vi "Draw Staff.vi"(4 "Line Spacing":i16=30, 6 "Line Length":i16=600, 9 "Start y":i16=200, 10 "Start x":i16=80, 11 "picture in":picture) -> (1 "End y":i16=230, 3 "picture out":picture)   [LabVIEW 2014]
panel:
  in  "y":i16=-120
  in  "x":i16
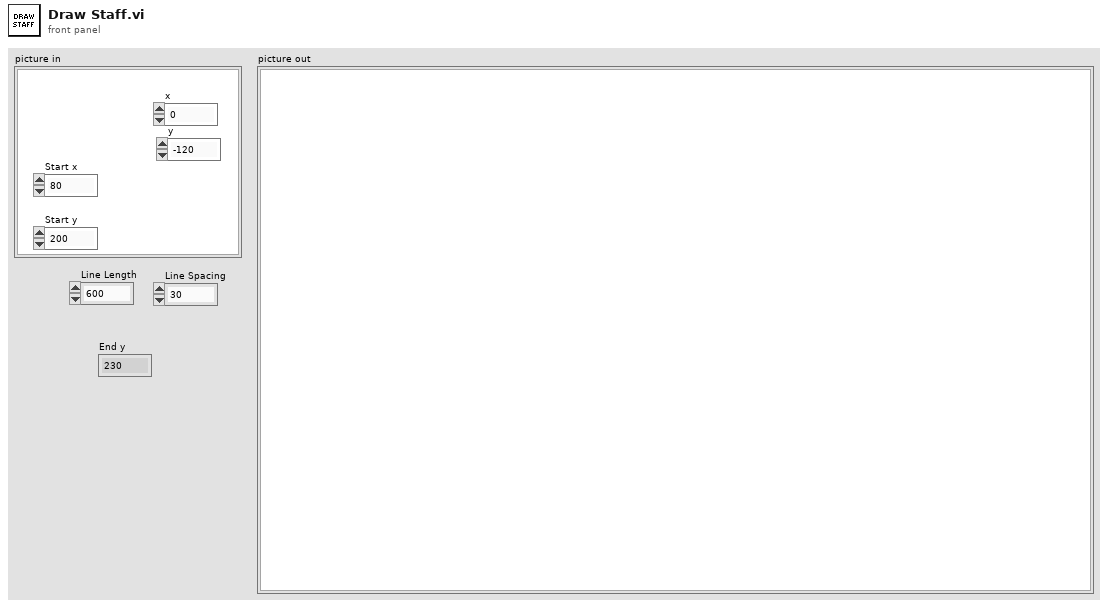
[diagram p1: front panel]
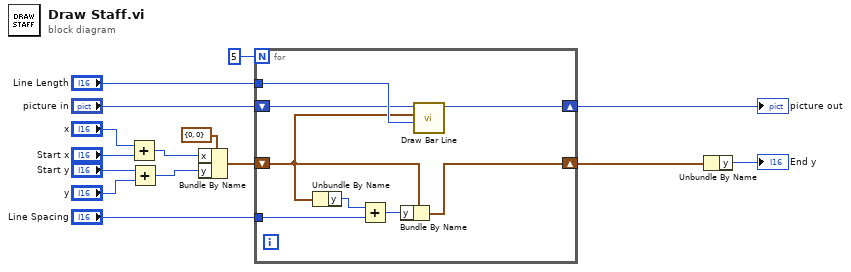
[diagram p0: block diagram]
diagram:
  n1 = Add(x="x", y="Start x") -> (x+y=w4:i16)
  n2 = Add(x="Start y", y="y") -> (x+y=w5:i16)
  n3 = Bundle By Name(cluster=cluster{"x":i16, "y":i16} {"x"=0, "y"=0} ("end point"), "x"=w4, "y"=w5) -> (w15:cluster{"x":i16, "y":i16})
  n4 = for {
    N: 5 -> [_]
    tunnel: "Line Length" -> [w23]
    tunnel: "Line Spacing" -> [w20]
    shift-right: [w18] -> w2
    shift-left: "picture in" -> [w17]
    shift-right: [w19] -> w12
    shift-left: w15 -> [w16]
    n5 = Unbundle By Name(w16) -> ("y"=w22:i16)
    n6 = Add(x=w22, y=w20) -> (x+y=w21:i16)
    n7 = Bundle By Name(cluster=w16, "y"=w21) -> (w19:cluster{"x":i16, "y":i16})
    n8 = call "Draw Bar Line.vi"("Line Length"=w23, "end point"=w16, "picture in"=w17) -> ("picture out"=w18:picture)  [unwired: 8 in]
  }
  "picture out" <- w2
  n9 = Unbundle By Name(w12) -> ("y"=→"End y":i16)
